vi "HWT_UNITHERM_Proc_Commands.vi"(8 "error in (no error)":errorcluster, 10 "Settings":T1, 11 "Queue in":refnum<queue>) -> (0 "error out":errorcluster)   [LabVIEW 2015]
uses:
  Core/Process/Uni-Therm/VIs/HWT_UNITHERM_Proc_Globals.vi
  Core/Process/_Shared/HWT_Shared_Proc_Globals.vi
  Controls/Control_General Command Cluster.ctl
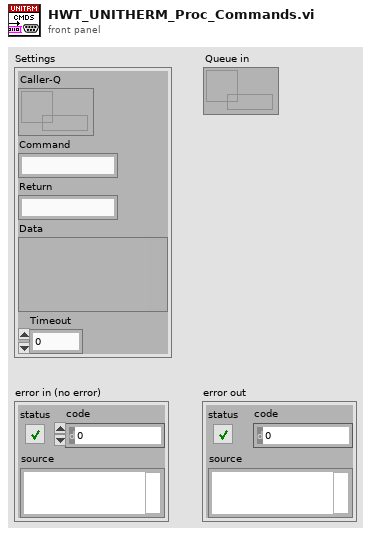
[diagram p1: front panel]
types:
  T1 = typedef "Control_General Command Cluster.ctl" = cluster{"Caller-Q":refnum<queue>, "Command":string, "Return":string, "Data":variant, "Timeout":dbl}
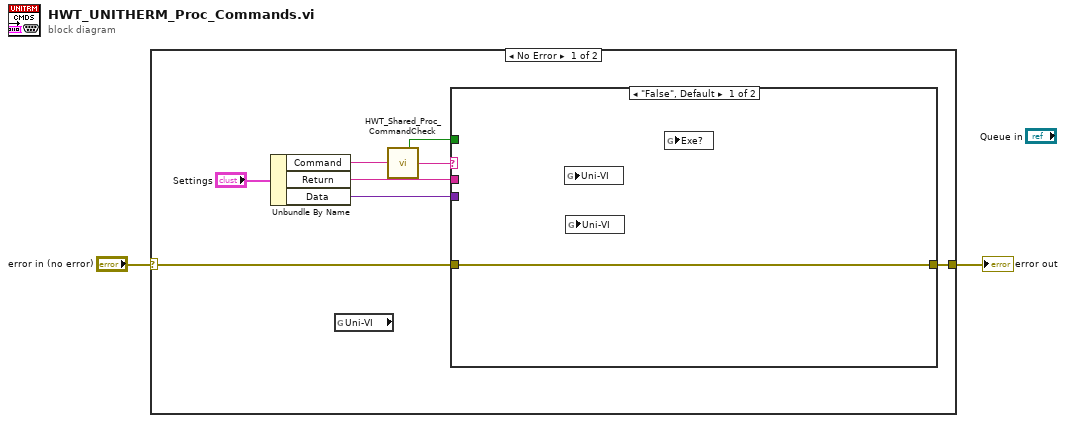
[diagram p0: block diagram]
diagram:
  n1 = case shown="No Error" "error in (no error)" {
    selector: "error in (no error)" -> [w3 w13]
    tunnel: [w4 w13] -> w2
    frame No Error {
      n2 = Unbundle By Name("Settings") -> ("Command"=w9:string, "Return"=w6:string, "Data"=w5:variant)
      n3 = global read "HWT_UNITHERM_Proc_Globals.vi" "Uni-VI"() -> ()  [unwired: 1 out]
      n4 = call "HWT_Shared_Proc_CommandCheck.vi"("Cmd In"=w9) -> ("Local?"=w7:bool, "Cmd Out"=w8:string)  [unwired: 13 in]
      n5 = case shown="\"False\", Default" w8 {
        tunnel: w7 -> [_ _]
        tunnel: w6 -> [_ _]
        tunnel: w5 -> [_ _]
        tunnel: w3 -> [w11 w12]
        tunnel: [w11 w12] -> w4
        frame "False", Default {
          n6 = global read "HWT_UNITHERM_Proc_Globals.vi" "Uni-VI"() -> ()  [unwired: 1 in]
          n7 = global read "HWT_UNITHERM_Proc_Globals.vi" "Uni-VI"() -> ()  [unwired: 1 in]
          n8 = global read "HWT_Shared_Proc_Globals.vi" "Exe?"() -> ()  [unwired: 1 in]
        }
        frame "True" {
        }
      }
    }
    frame Error {
    }
  }
  "error out" <- w2
